vi "RemoveUnderscores.vi"(9 "Extension":string=".*", 11 "Filenames In":string[](array[string])) -> (3 "Filenames Out":string[](array[string]))   [LabVIEW 2024]
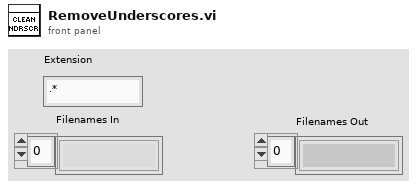
[diagram p1: front panel]
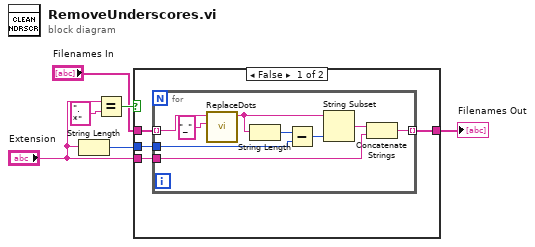
[diagram p0: block diagram]
diagram:
  n1 = String Length(string="Extension") -> (length=w1:i32)
  n2 = Equal?(x="Extension", y=".*") -> (x = y?=w5:bool)
  n3 = case shown="False" w5 {
    tunnel: "Filenames In" -> [w10 w20]
    tunnel: "Extension" -> [w9 _]
    tunnel: [w8 w20] -> w3
    tunnel: w1 -> [w7 _]
    frame False {
      n4 = for {
        tunnel: w10 -> [w17] mode=indexing
        tunnel: w9 -> [w19]
        tunnel: [w18] -> w8 mode=indexing
        tunnel: w7 -> [w16]
        n5 = call "ReplaceDots.vi"("search string"="_", "String In"=w17) -> ("String Out"=w13:string)  [unwired: 8 in, 1 out]
        n6 = String Length(string=w13) -> (length=w15:i32)
        n7 = Subtract(x=w15, y=w16) -> (x-y=w14:i32)
        n8 = String Subset(string=w13, length (rest)=w14) -> (substring=w12:string)  [unwired: 1 in]
        n9 = Concatenate Strings(w12, w19) -> (w18:string)
      }
    }
    frame True {
    }
  }
  "Filenames Out" <- w3
